vi "Auto Calibrate.vi"(8 "error in (no error)":errorcluster, 11 "MSOX6004 in":refnum<class "MSOX6004.lvclass">) -> (0 "error out":errorcluster, 2 "Cal Passed ? (T:Yes)":bool, 3 "MSOX6004 out":refnum<class "MSOX6004.lvclass">)   [LabVIEW 2018, in "MSOX6004.lvlib" / "MSOX6004.lvclass"]
doc: "This Override method is used to call the Auto-Calibrate function of the Oscope instrument. The boolean output 'Cal Passed? (T:Yes)' carries out the auto-calibration result."
uses:
  MSOX6004.lvclass
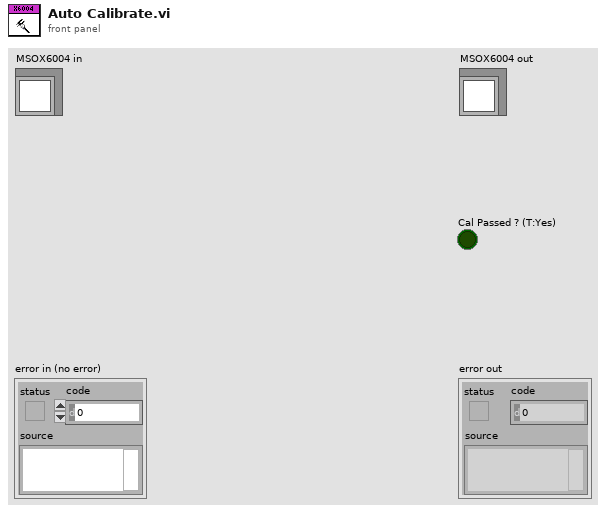
[diagram p1: front panel]
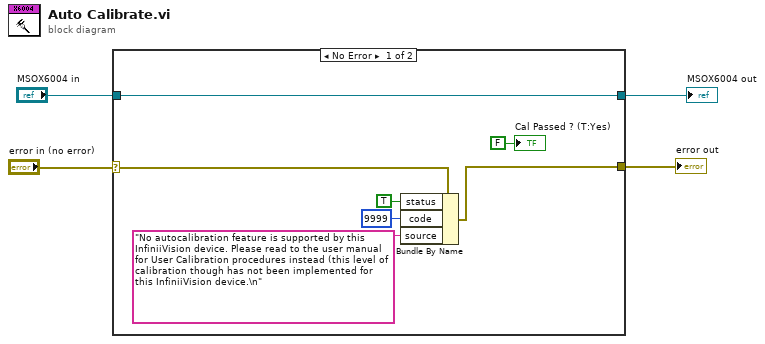
[diagram p0: block diagram]
diagram:
  n1 = case shown="No Error" "error in (no error)" {
    selector: "error in (no error)" -> [w11 w12]
    tunnel: "MSOX6004 in" -> [w8 w13]
    tunnel: [w8 w13] -> w2
    tunnel: [w5 w12] -> w1
    frame No Error {
      n2 = Bundle By Name(cluster=w11, "status"=TRUE, "code"=9999, "source"="No autocalibration feature is supported by this InfiniiVision device. Please read to the user manual for User Calibration procedures instead (this level of calibration though has not been implemented for this InfiniiVision device.\n") -> (w5:errorcluster)
      "Cal Passed ? (T:Yes)" <- FALSE ("Cal Passed ? (T:Yes)")
    }
    frame Error {
    }
  }
  "error out" <- w1
  "MSOX6004 out" <- w2
